vi "CALC_MARK_FUNC_DOM_USER_STOP.vi"(0 "VISA IN":refnum<visa-resource-name>, 1 "Marker number":i32, 2 "Stop Value":i32, 5 "error in":errorcluster, 7 "Channel":i32) -> (14 "VISA Out":refnum<visa-resource-name>, 19 "error out":errorcluster)   [LabVIEW 2018, in "PNA-X.lvlib"]
doc: "CALCulate<cnum>:MARKer<mkr>:FUNCtion:DOMain:USER:STOP <stop> \n(Read-Write) Sets the stop of the span that the marker's x-axis travel will be constrained to. \nUse CALC:MARK:FUNC:DOM:USER<range> to set range number \nUse CALC:MARK:FUNC:DOM:USER:STARt to set the stop value. \nNote: If the marker is assigned to range 0 (full span), the USER:STARt and STOP commands \ngenerate an error. You cannot set the STARt and STOP values for \"Full Span\". \nNote: This command does the same as CALC:FUNC:DOM:USER:STOP \nSee Critical Note \nParameters \n1535\n\n<cnum> Channel number of the measurement. There must be a selected measurement on that \nchannel. If unspecified, <cnum> is set to 1. \n<mkr> Any marker number from 1 to 10; if unspecified, value is set to 1. \n<stop> Stop value of x-axis span; Choose any number between the analyzer's MINimum and \nMAXimum x-axis value. \nExamples CALC:MARK:FUNC:DOM:USER:STOP 500e6 \ncalculate2:marker8:function:domain1:user:stop 1e12 \nQuery \nSyntax"
uses:
  PNA-X.lvlib
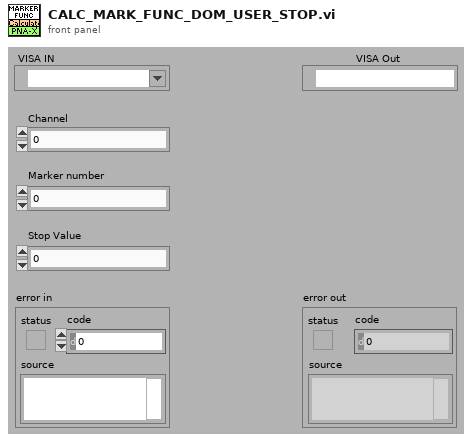
[diagram p1: front panel]
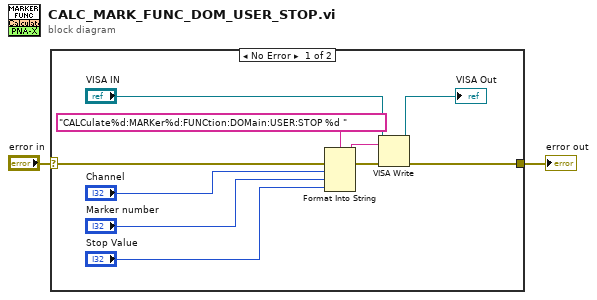
[diagram p0: block diagram]
diagram:
  n1 = case shown="No Error" "error in" {
    selector: "error in" -> [w12 w13]
    tunnel: [w7 w13] -> w1
    frame No Error {
      n2 = Format Into String(format string="CALCulate%d:MARKer%d:FUNCtion:DOMain:USER:STOP %d " ("Cmdline"), error in=w12, "Channel", "Marker number", "Stop Value") -> (resulting string=w10:string, error out=w11:errorcluster)  [unwired: 1 in]
      n3 = VISA Write(VISA resource name="VISA IN", write buffer=w10, error in (no error)=w11) -> (VISA resource name out=→"VISA Out":refnum<visa-resource-name>, error out=w7:errorcluster)  [unwired: 1 out]
    }
    frame Error {
    }
  }
  "error out" <- w1
